vi "Lift Set Motors.vi"(8 "error in (no error)":errorcluster, 10 "Motor output":dbl, 11 "Motors in":T10) -> (0 "error out":errorcluster, 3 "Motors out":T10)   [LabVIEW 2014]
uses:
  <vilib>/Rock Robotics/WPI/MotorControl/WPI_MotorControlDeviceRef.ctl
  <vilib>/Rock Robotics/WPI/MotorControl/WPI_MotorControlType.ctl
  <vilib>/Rock Robotics/SystemInterfaces/Typedef/FPGA_TypedefDigitalModule.ctl
  <vilib>/Rock Robotics/SystemInterfaces/DIO/FPGA_DIOPWMChannel.ctl
  <vilib>/Rock Robotics/WPI/PWM/WPI_PWMDeadband.ctl
  <vilib>/Rock Robotics/WPI/CAN/Jaguar/SubVIs/WPI_CANJaguar_ControlMode.ctl
  <vilib>/Rock Robotics/WPI/CAN/TalonSRX/WPI_CANTalonSRX_APIControlMode.ctl
  <vilib>/Rock Robotics/WPI/PWM/WPI_PWMTransform_ConPane.ctl
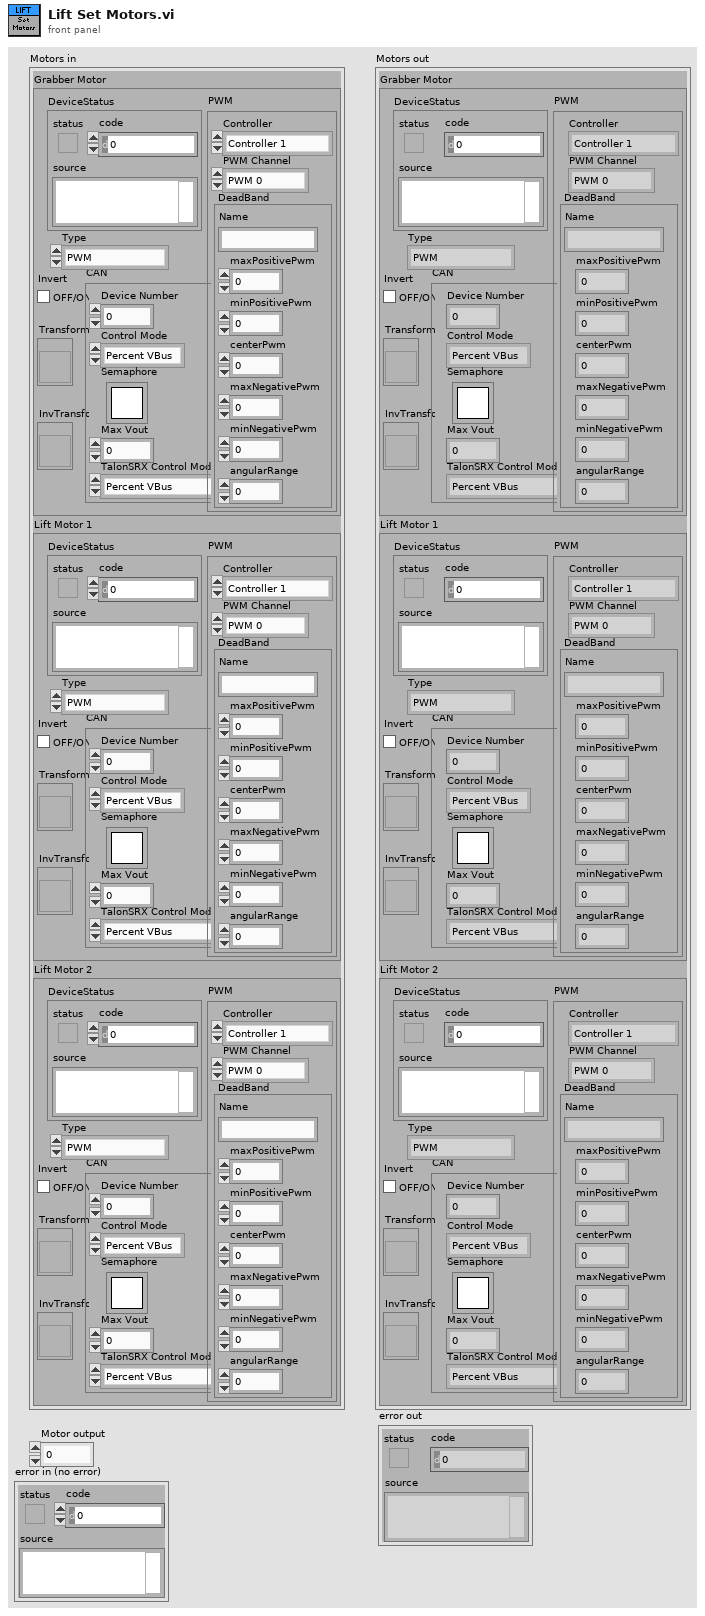
[diagram p1: front panel]
types:
  T1 = typedef "WPI_MotorControlDeviceRef.ctl" = cluster{"DeviceStatus":errorcluster, "Type":T2, "PWM":cluster{"Controller":T3, "PWM Channel":T4, "DeadBand":T5}, "CAN":cluster{"Device Number":u8, "Control Mode":T6, "Semaphore":T7, "Max Vout":dbl, "TalonSRX Control Mode":T8}, "Invert":bool, "TransformRef":T9, "InvTransformRef":T9}
  T2 = typedef "WPI_MotorControlType.ctl" = enum16{"PWM", "CAN", "CANTalonSRX"}
  T3 = typedef "FPGA_TypedefDigitalModule.ctl" = enum16{"Controller 1"}
  T4 = typedef "FPGA_DIOPWMChannel.ctl" = enum8{"PWM 0", "PWM 1", "PWM 2", "PWM 3", "PWM 4", "PWM 5", "PWM 6", "PWM 7", "PWM 8", "PWM 9", "PWM MXP 0", "PWM MXP 1", "PWM MXP 2", "PWM MXP 3", "PWM MXP 4", "PWM MXP 5", "PWM MXP 6", "PWM MXP 7", "PWM MXP 8", "PWM MXP 9", "Invalid"}
  T5 = typedef "WPI_PWMDeadband.ctl" = cluster{"Name":string, "maxPositivePwm":i32, "minPositivePwm":i32, "centerPwm":i32, "maxNegativePwm":i32, "minNegativePwm":i32, "angularRange":u16}
  T6 = typedef "WPI_CANJaguar_ControlMode.ctl" = enum8{"Percent VBus", "Current", "Speed", "Position", "Voltage"}
  T7 = typedef "Semaphore RefNum" = refnum<k1>
  T8 = typedef "WPI_CANTalonSRX_APIControlMode.ctl" = enum8{"Percent VBus", "Speed", "Position", "Slave", "Unchanged / Invalid"}
  T9 = typedef "WPI_PWMTransform_ConPane.ctl" = refnum<vi>
  T10 = cluster{"Grabber Motor":T1, "Lift Motor 1":T1, "Lift Motor 2":T1}
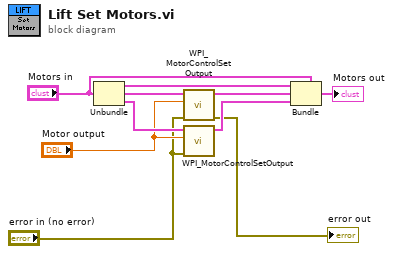
[diagram p0: block diagram]
diagram:
  n1 = Unbundle("Motors in") -> ("Grabber Motor"=w8:T1, "Lift Motor 1"=w9:T1, "Lift Motor 2"=w10:T1)
  n2 = call <vilib>:"WPI_MotorControlSetOutput.vi"("error in (no error)"="error in (no error)", "Output"="Motor output", "MotorControlDevRef"=w9) -> ("error out"=→"error out":errorcluster, "MotorControlDevRef"=w4:T1)  [unwired: 6 in, 1 out]
  n3 = call <vilib>:"WPI_MotorControlSetOutput.vi"("error in (no error)"="error in (no error)", "Output"="Motor output", "MotorControlDevRef"=w10) -> ("MotorControlDevRef"=w5:T1)  [unwired: 6 in, 2 out]
  n4 = Bundle(cluster="Motors in", "Grabber Motor"=w8, "Lift Motor 1"=w4, "Lift Motor 2"=w5) -> (→"Motors out":T10)
